vi "Query Capabilities (Range).vi"(0 "VISA resource name":refnum<visa-resource-name>, 5 "Absolute Maximums (T)":bool=TRUE, 11 "error in (no error)":errorcluster) -> (4 "VISA resource name out":refnum<visa-resource-name>, 6 "Number of Ranges":u32 max=12 step=1, 15 "error out":errorcluster)   [LabVIEW 2012, in "NH Research Regenerative Test Series.lvlib"]
doc: "This query will retrieve the number of ranges for the Module."
uses:
  <instrlib>/NH Research Regenerative Test Series/NH Research Regenerative Test Series.lvlib
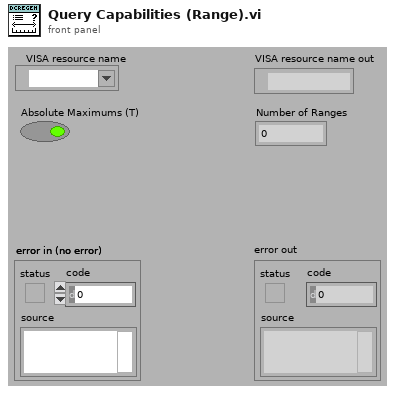
[diagram p1: front panel]
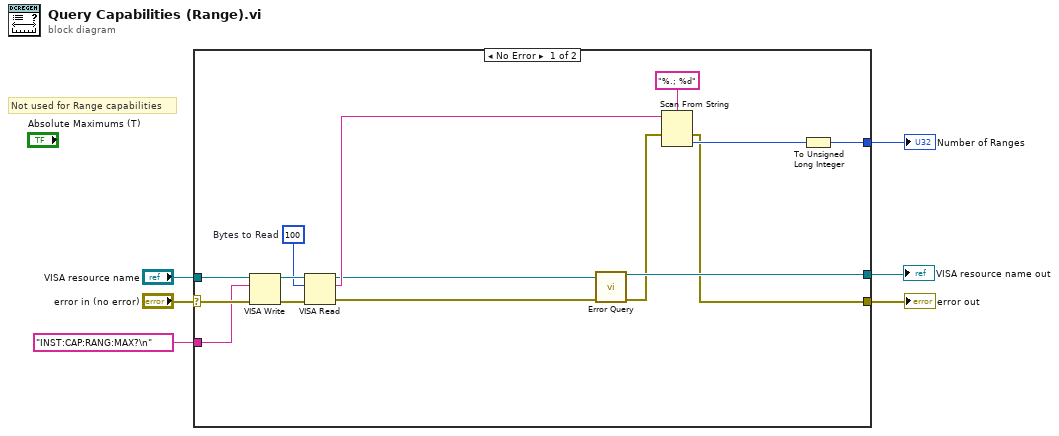
[diagram p0: block diagram]
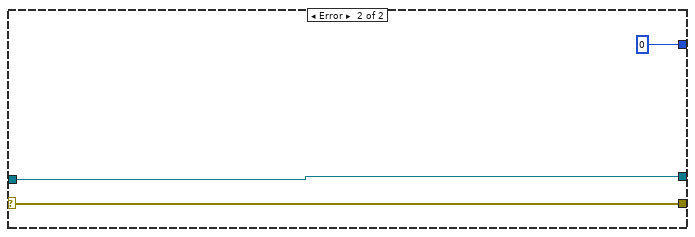
[diagram p2: hidden frame]
diagram:
  # "Not used for Range capabilities"
  n1 = case shown="No Error" "error in (no error)" {
    selector: "error in (no error)" -> [w19 w24]
    tunnel: [w9 w24] -> w5
    tunnel: [w17 w23] -> w3
    tunnel: "VISA resource name" -> [w18 w23]
    tunnel: [w14 u32 0] -> w2
    tunnel: "INST:CAP:RANG:MAX?\n" ("write buffer") -> [w13 _]
    frame No Error {
      w12 = u32 100  # Bytes to Read
      n2 = VISA Write(VISA resource name=w18, write buffer=w13, error in (no error)=w19) -> (VISA resource name out=w20:refnum<visa-resource-name>, error out=w21:errorcluster)  [unwired: 1 out]
      n3 = VISA Read(VISA resource name=w20, byte count=w12, error in (no error)=w21) -> (VISA resource name out=w8:refnum<visa-resource-name>, read buffer=w10:string, error out=w7:errorcluster)  [unwired: 1 out]
      n4 = call <instrlib>:"Error Query.vi"("VISA resource name"=w8, "error in (no error)"=w7) -> ("VISA resource name out"=w17:refnum<visa-resource-name>, "error out"=w16:errorcluster)  [unwired: 10 in, 2 out]
      n5 = Scan From String(format string="%.; %d", input string=w10, error in=w16) -> (error out=w9:errorcluster, output 1=w15:i32)  [unwired: 2 in, 2 out]
      n6 = To Unsigned Long Integer(number=w15) -> (unsigned 32bit integer=w14:u32)
    }
    frame Error {
    }
  }
  "error out" <- w5
  "VISA resource name out" <- w3
  "Number of Ranges" <- w2
